vi "Octal Channel Engine.vi"(0 "Notifier Name":string) -> ()   [LabVIEW 2016]
uses:
  AOTF Controls/AOTF Actions.ctl
  AOTF Controls/AOTF Notifier Element.ctl
  Octal Channel Type Defs/Octal Channel AOTF Config.ctl
panel:
  in  "Wavelength (nm)":u16(ring)
  in  "Line On/Off":bool
  out "Controller Response":string
  in  "Blank All":bool
  in  "Quit":bool
  in  "Power (%)":dbl
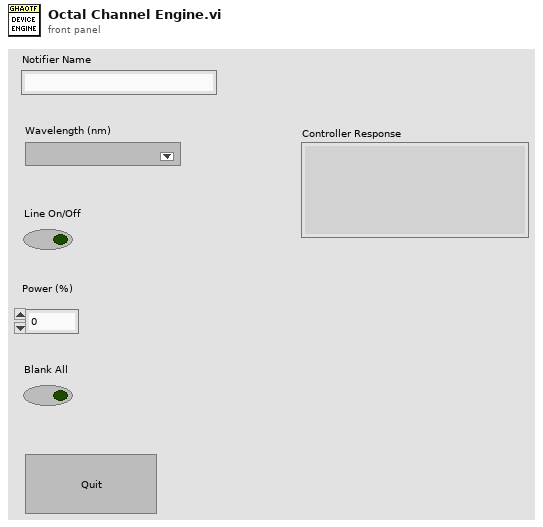
[diagram p1: front panel]
types:
  T1 = typedef "AOTF Notifier Element.ctl" = cluster{"AOTF Action":T2, "Laser Line":string, "Power (%)":dbl, "Beam Blank On/Off":bool, "Line On/Off":bool, "Error":errorcluster, "Wavelengths (nm)":string[]}
  T2 = typedef "AOTF Actions.ctl" = enum16{"Error Check", "Blank", "Line On/Off", "Set Power", "Status", "Quit"}
  T3 = typedef "Octal Channel AOTF Config.ctl" = cluster{"Wavelength (nm)":u16[], "Channel Number":u8[], "Frequency (MHz)":dbl[], "Max Power":u16[]}
  T4 = enum32{"Invalid", "Standard", "Closed", "Hidden", "Minimized", "Maximized"}
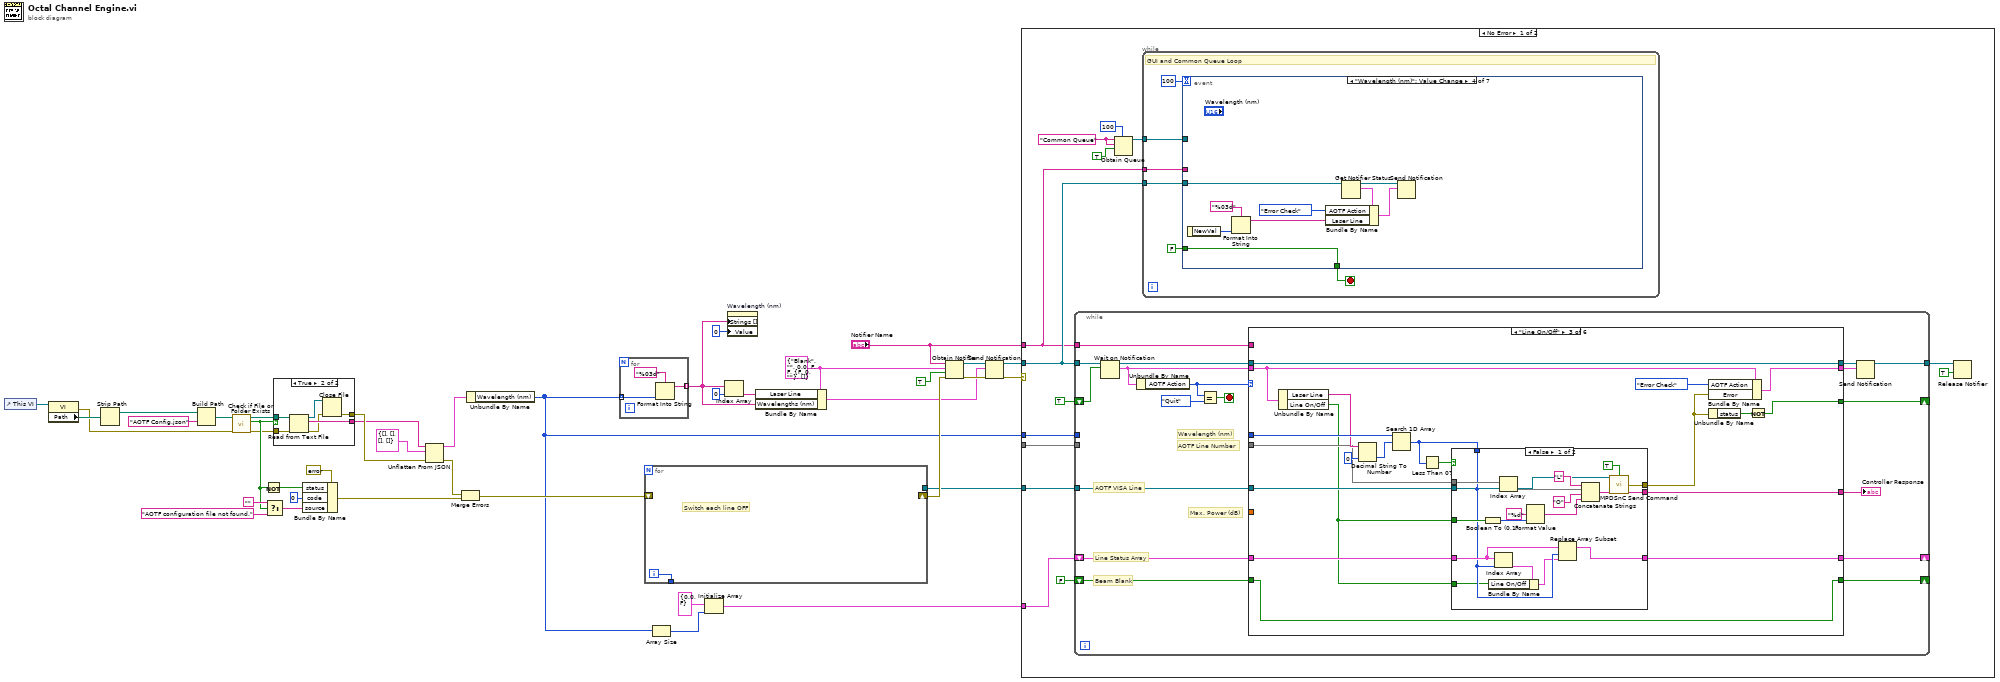
[diagram p0: block diagram]
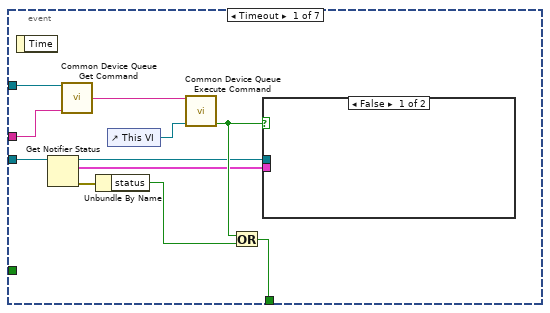
[diagram p2: hidden frame]
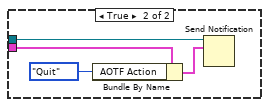
[diagram p3: hidden frame]
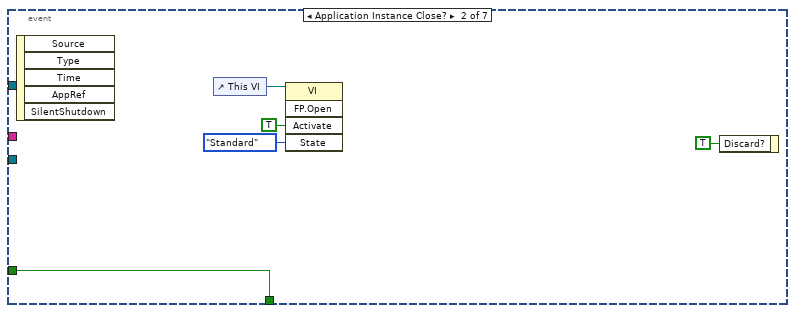
[diagram p4: hidden frame]
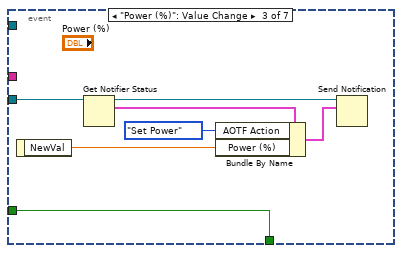
[diagram p5: hidden frame]
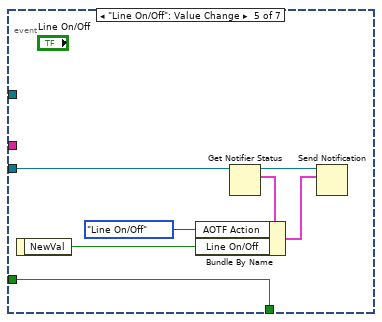
[diagram p6: hidden frame]
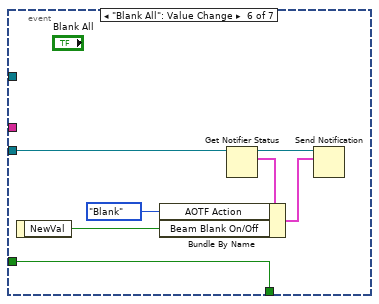
[diagram p7: hidden frame]
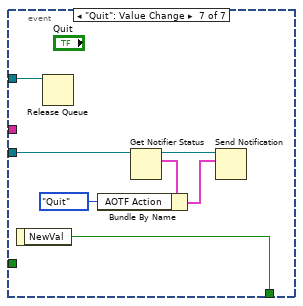
[diagram p8: hidden frame]
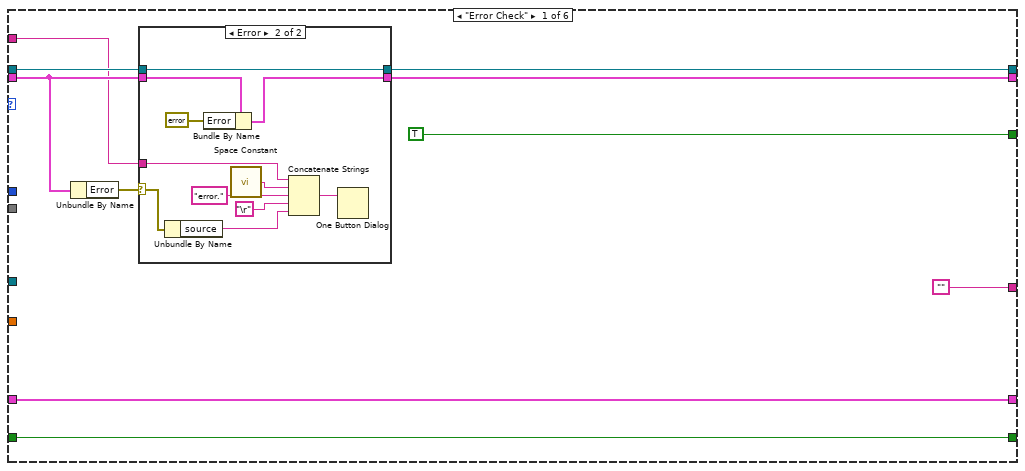
[diagram p9: hidden frame]
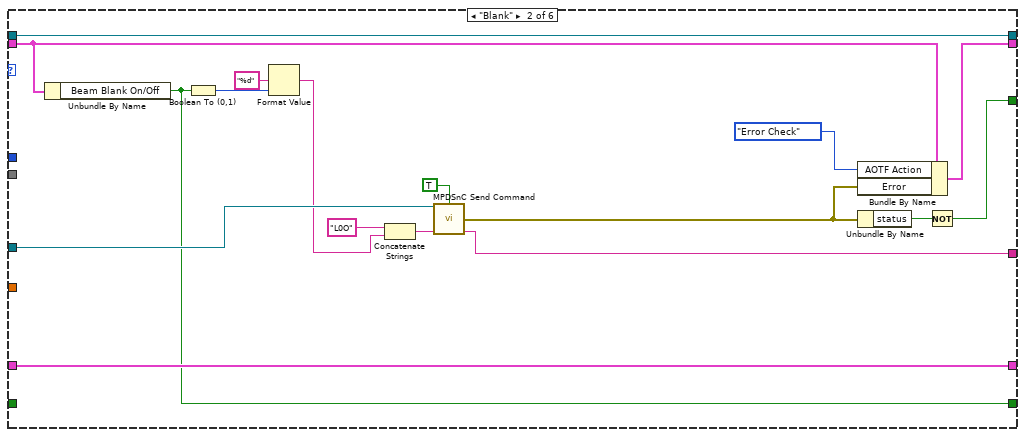
[diagram p11: hidden frame]
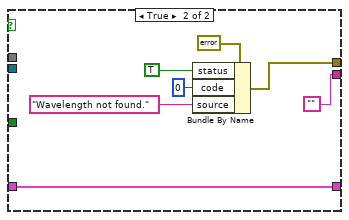
[diagram p12: hidden frame]
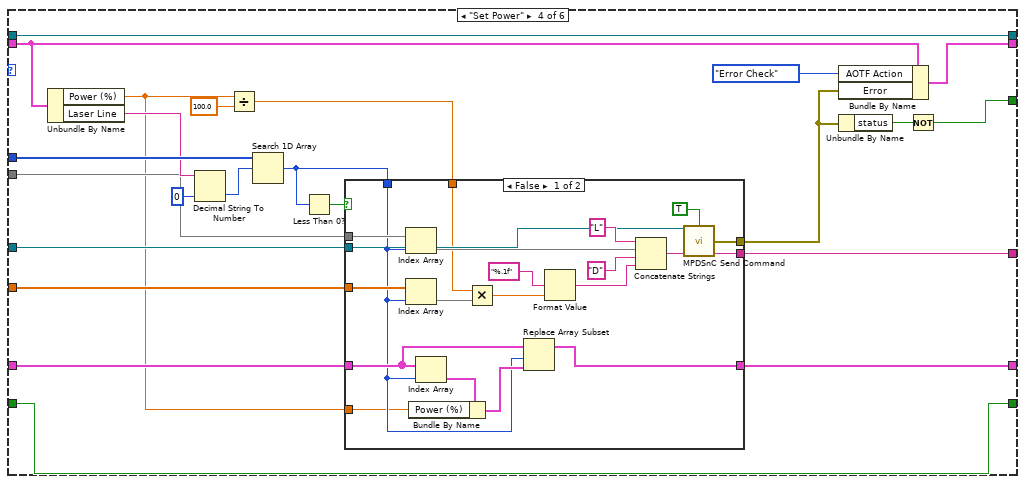
[diagram p13: hidden frame]
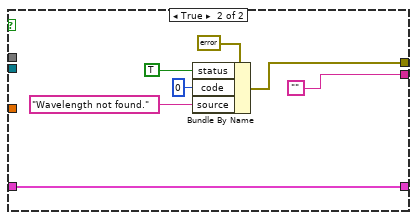
[diagram p14: hidden frame]
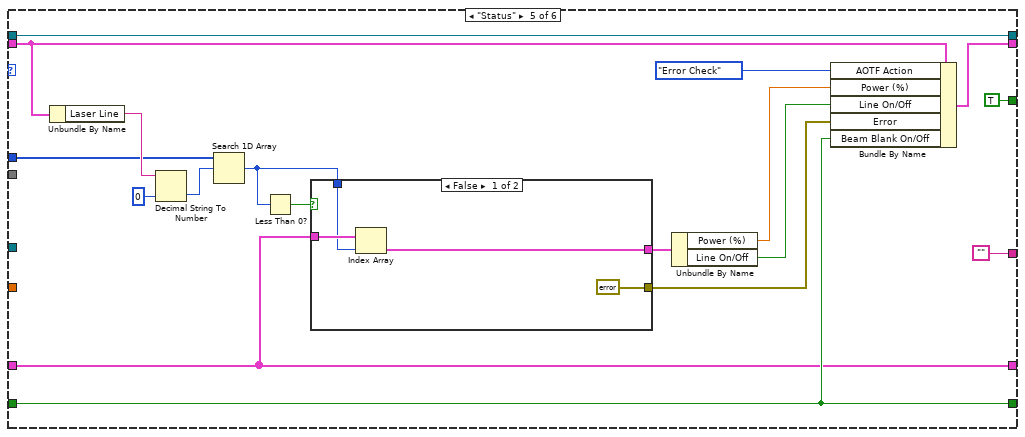
[diagram p15: hidden frame]
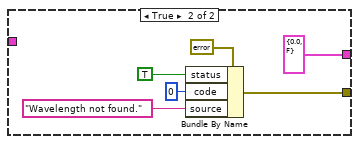
[diagram p16: hidden frame]
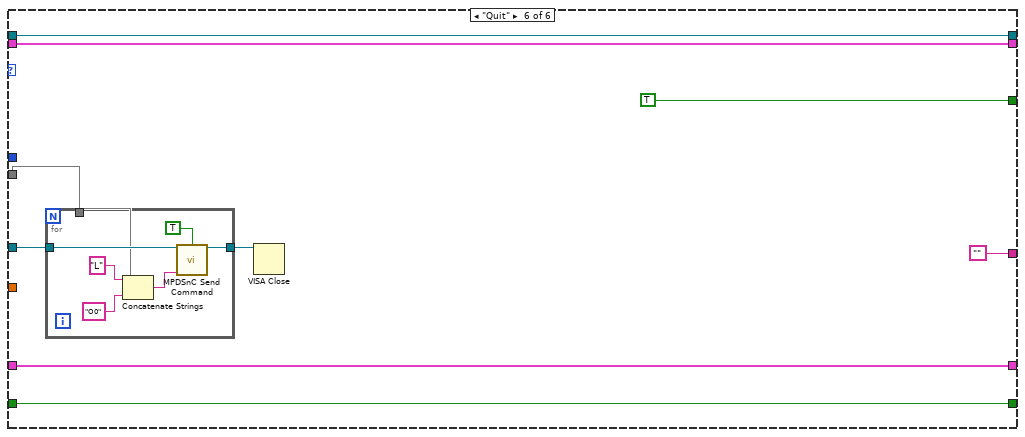
[diagram p17: hidden frame]
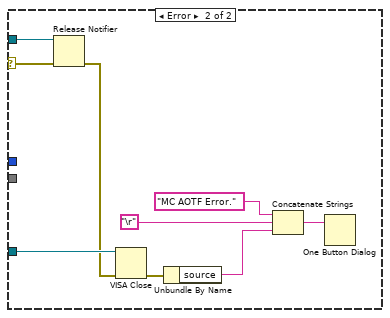
[diagram p18: hidden frame]
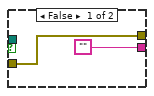
[diagram p19: hidden frame]
diagram:
  w10 = T1 {"AOTF Action"=enum."Blank", "Laser Line"="", "Power (%)"=0.0, "Beam Blank On/Off"=FALSE, "Line On/Off"=FALSE, "Error"={"status"=FALSE, "code"=0, "source"=""}, "Wavelengths (nm)"=[]} ("AOTFQueueCtrl")
  n1 = control-ref of="This VI"() -> (w40:refnum<vi>)
  n2 = property class="VI"(reference=w40) -> (error out=w27:errorcluster, "Path"=w39:path)  [unwired: 1 in, 1 out]
  n3 = Strip Path(path=w39) -> (stripped path=w38:path)  [unwired: 1 out]
  n4 = Build Path(base path=w38, name or relative path="AOTF Config.json") -> (appended path=w36:path)
  n5 = call <vilib>:"Check if File or Folder Exists.vi"("error in (no error)"=w27, "path"=w36) -> ("error out"=w26:errorcluster, "file or folder exists?"=w29:bool, "dup path"=w28:path)  [unwired: 7 in]
  n6 = Not(x=w29) -> (.not. x?=w34:bool)
  n7 = Select(t="", s=w29, f="AOTF configuration file not found." ("source")) -> (s? t:f=w30:string)
  n8 = case shown="True" w29 {
    tunnel: w28 -> [_ w48]
    tunnel: ["" w47] -> w22
    tunnel: w26 -> [w41 w45]
    tunnel: [w41 w43] -> w25
    frame False {
    }
    frame True {
      n9 = Read from Text File(file (use dialog)=w48, error in=w45) -> (refnum out=w46:refnum<file>, text=w47:string, error out=w44:errorcluster)  [unwired: 2 in, 1 out]
      n10 = Close File(refnum=w46, error in=w44) -> (error out=w43:errorcluster)  [unwired: 1 out]
    }
  }
  n11 = Bundle By Name(cluster=errorcluster {"status"=FALSE, "code"=0, "source"=""} ("Error"), "status"=w34, "code"=0, "source"=w30) -> (w23:errorcluster)
  n12 = Unflatten From JSON(JSON string=w22, type and defaults=T3 {"Wavelength (nm)"=[], "Channel Number"=[], "Frequency (MHz)"=[], "Max Power"=[]} ("AOTF Config"), error in (no error)=w25) -> (value=w7:T3, error out=w24:errorcluster)  [unwired: 4 in]
  n13 = Merge Errors(w24, w23) -> (w8:errorcluster)
  n14 = Unbundle By Name(w7) -> ("Wavelength (nm)"=w6:u16[])
  n15 = for {
    tunnel: w6 -> [w51] mode=indexing
    tunnel: [w50] -> w4 mode=indexing
    n16 = Format Into String(format string="%03d", w51) -> (resulting string=w50:string)  [unwired: 2 in, 1 out]
  }
  n17 = for {
    tunnel: [_] -> w17
    shift-right: [_] -> w20
    shift-left: w8 -> [_]
    tunnel: [w52] -> _
    i -> [w52]
    # "Switch each line OFF"
  }
  n18 = Array Size(array=w6) -> (size(s)=w5:i32)
  n19 = Initialize Array(cluster{"Power (%)":dbl, "Line On/Off":bool} {"Power (%)"=0.0, "Line On/Off"=FALSE} ("Line Staus Cluster"), w5) -> (w15:cluster{"Power (%)":dbl, "Line On/Off":bool}[])
  n20 = Index Array(array=w4, index=0) -> (element=w2:string)
  n21 = property on="Wavelength (nm)" class="Ring (strict)"("Strings []"=w4, "Value"=u16 0 ("index")) -> ()  [unwired: 2 in, 2 out]
  n22 = Bundle By Name(cluster=w10, "Laser Line"=w2, "Wavelengths (nm)"=w4) -> (w9:T1)
  n23 = Obtain Notifier(name (unnamed)="Notifier Name", notification data type=w10, create if not found? (T)=TRUE, error in (no error)=w20) -> (notifier out=w14:refnum<notifier>, error out=w13:errorcluster)  [unwired: 1 out]
  n24 = Send Notification(notification=w9, notifier=w14, error in (no error)=w13) -> (notifier out=w12:refnum<notifier>, error out=w11:errorcluster)
  n25 = case shown="No Error" w11 {
    selector: w11 -> [_ w336]
    tunnel: w12 -> [w62 w337]
    tunnel: "Notifier Name" -> [w58 _]
    tunnel: w6 -> [w57 _]
    tunnel: _ -> [w56 _]
    tunnel: w17 -> [w55 w331]
    tunnel: w15 -> [w54 _]
    frame No Error {
      w66 = "Common Queue" ("Unique Notifier Name")
      n26 = while {
        tunnel: w62 -> [w147]
        shift-right: [w138] -> _
        shift-left: TRUE ("ignore previous (F)") -> [w146]
        tunnel: [w137] -> w60
        tunnel: w58 -> [w136]
        tunnel: w57 -> [_]
        tunnel: w56 -> [_]
        tunnel: w55 -> [w135]
        shift-right: [w130] -> _
        shift-left: w54 -> [w133]
        shift-right: [w131] -> _
        shift-left: FALSE -> [w132]
        stop <- w141 stop-if-true
        # "Wavelength (nm)"
        # "AOTF Line Number"
        # "Line Status Array"
        # "Beam Blank"
        # "AOTF VISA Line"
        # "Max. Power (dB)"
        n27 = Wait on Notification(notifier=w147, ignore previous (F)=w146) -> (notifier out=w145:refnum<notifier>, notification=w144:T1)  [unwired: 2 in, 2 out]
        n28 = Unbundle By Name(w144) -> ("AOTF Action"=w143:T2)
        n29 = Equal?(x=w143, y=AOTF_Actions."Quit") -> (x = y?=w141:bool)
        n30 = case shown="\"Line On/Off\"" w143 {
          tunnel: w145 -> [w157 w187 w203 w256 w301 w321]
          tunnel: w144 -> [w155 w186 w205 w252 w296 w320]
          tunnel: [w153 w187 w203 w256 w301 w321] -> w140
          tunnel: [w152 w185 w204 w251 w292 w320] -> w139
          tunnel: [TRUE w182 w192 w250 TRUE TRUE] -> w138
          tunnel: w136 -> [w154 _ _ _ _ _]
          tunnel: _ -> [_ _ w200 w247 w297 _]
          tunnel: _ -> [_ _ w197 w243 _ w315]
          tunnel: _ -> [_ _ _ w240 _ _]
          tunnel: w135 -> [_ w180 w196 w239 _ w314]
          tunnel: ["" w173 w194 w238 "" ""] -> w134
          tunnel: w133 -> [w149 w172 w191 w237 w285 w317]
          tunnel: w132 -> [w148 _ w189 w234 w286 w316]
          tunnel: [w148 w171 w189 w234 w286 w316] -> w131
          tunnel: [w149 w172 w190 w235 w285 w317] -> w130
          frame "Error Check" {
            n31 = Unbundle By Name(w155) -> ("Error"=w156:errorcluster)
            n32 = case shown="Error" w156 {
              selector: w156 -> [_ w163]
              tunnel: w155 -> [w158 w167]
              tunnel: [w159 w165] -> w153
              tunnel: w157 -> [w159 w165]
              tunnel: w154 -> [_ w162]
              tunnel: [w158 w164] -> w152
              frame No Error {
              }
              frame Error {
                n33 = Unbundle By Name(w163) -> ("source"=w161:string)
                n34 = Bundle By Name(cluster=w167, "Error"=errorcluster {"status"=FALSE, "code"=0, "source"=""}) -> (w164:T1)
                n35 = call <vilib>:"Space Constant.vi"() -> ("String"=w170:string)
                n36 = Concatenate Strings(w162, w170, "error." ("string"), "\r", w161) -> (w168:string)
                n37 = One Button Dialog(message=w168) -> ()  [unwired: 1 in, 1 out]
              }
            }
          }
          frame "Blank" {
            n38 = Unbundle By Name(w186) -> ("Beam Blank On/Off"=w171:bool)
            n39 = Boolean To (0,1)(Boolean=w171) -> (0, 1=w176:i16)
            n40 = Format Value(format string="%d", value (0)=w176) -> (output string=w174:string)  [unwired: 1 in]
            n41 = Concatenate Strings("L0O", w174) -> (w177:string)
            n42 = call "MPDSnC Send Command.vi"("VISA Ref"=w180, "Wait for Reply?"=TRUE, "Command"=w177) -> ("Error Out"=w181:errorcluster, "Response"=w173:string)  [unwired: 10 in, 1 out]
            n43 = Bundle By Name(cluster=w186, "AOTF Action"=AOTF_Actions."Error Check", "Error"=w181) -> (w185:T1)
            n44 = Unbundle By Name(w181) -> ("status"=w183:bool)
            n45 = Not(x=w183) -> (.not. x?=w182:bool)
          }
          frame "Line On/Off" {
            n46 = Unbundle By Name(w205) -> ("Laser Line"=w199:string, "Line On/Off"=w188:bool)
            n47 = Decimal String To Number(string=w199, default (0L)=u16 0 ("default (0 I32)")) -> (number=w202:u16)  [unwired: 1 in, 1 out]
            n48 = Search 1D Array(1D array=w200, element=w202) -> (index of element=w195:i32)  [unwired: 1 in]
            n49 = Less Than 0?(x=w195) -> (x < 0?=w198:bool)
            n50 = case shown="False" w198 {
              tunnel: w197 -> [w226 _]
              tunnel: [w221 w229] -> w193
              tunnel: w195 -> [w211 _]
              tunnel: w196 -> [w219 _]
              tunnel: [w218 ""] -> w194
              tunnel: w188 -> [w215 _]
              tunnel: w191 -> [w213 w227]
              tunnel: [w212 w227] -> w190
              tunnel: w188 -> [w208 _]
              frame False {
                n51 = Boolean To (0,1)(Boolean=w215) -> (0, 1=w217:i16)
                n52 = Index Array(array=w213, index=w211) -> (element=w210:cluster{"Power (%)":dbl, "Line On/Off":bool})
                n53 = Bundle By Name(cluster=w210, "Line On/Off"=w208) -> (w209:cluster{"Power (%)":dbl, "Line On/Off":bool})
                n54 = Index Array(array=w226, index=w211) -> (element=w225)
                n55 = Format Value(format string="%d", value (0)=w217) -> (output string=w214:string)  [unwired: 1 in]
                n56 = Replace Array Subset(array=w213, new element=w209, index=w211) -> (w212:cluster{"Power (%)":dbl, "Line On/Off":bool}[])
                n57 = Concatenate Strings("L", w225, "O", w214) -> (w222:string)
                n58 = call "MPDSnC Send Command.vi"("VISA Ref"=w219, "Wait for Reply?"=TRUE, "Command"=w222) -> ("Error Out"=w221:errorcluster, "Response"=w218:string)  [unwired: 10 in, 1 out]
              }
              frame True {
                n59 = Bundle By Name(cluster=errorcluster {"status"=FALSE, "code"=0, "source"=""} ("error out"), "status"=TRUE, "code"=0, "source"="Wavelength not found.") -> (w229:errorcluster)
              }
            }
            n60 = Bundle By Name(cluster=w205, "AOTF Action"=AOTF_Actions."Error Check", "Error"=w193) -> (w204:T1)
            n61 = Unbundle By Name(w193) -> ("status"=w206:bool)
            n62 = Not(x=w206) -> (.not. x?=w192:bool)
          }
          frame "Set Power" {
            n63 = Unbundle By Name(w252) -> ("Power (%)"=w236:dbl, "Laser Line"=w246:string)
            n64 = Decimal String To Number(string=w246, default (0L)=u16 0 ("default (0 I32)")) -> (number=w248:u16)  [unwired: 1 in, 1 out]
            n65 = Divide(x=w236, y=100.0) -> (x/y=w242:dbl)
            n66 = Search 1D Array(1D array=w247, element=w248) -> (index of element=w244:i32)  [unwired: 1 in]
            n67 = Less Than 0?(x=w244) -> (x < 0?=w245:bool)
            n68 = case shown="False" w245 {
              tunnel: w243 -> [w277 _]
              tunnel: [w270 w280] -> w241
              tunnel: w244 -> [w260 _]
              tunnel: w242 -> [w259 _]
              tunnel: w240 -> [w274 _]
              tunnel: w239 -> [w265 _]
              tunnel: [w264 ""] -> w238
              tunnel: w237 -> [w261 w278]
              tunnel: w236 -> [w258 _]
              tunnel: [w257 w278] -> w235
              frame False {
                n69 = Index Array(array=w277, index=w260) -> (element=w276)
                n70 = Index Array(array=w274, index=w260) -> (element=w272)
                n71 = Index Array(array=w261, index=w260) -> (element=w263:cluster{"Power (%)":dbl, "Line On/Off":bool})
                n72 = Bundle By Name(cluster=w263, "Power (%)"=w258) -> (w262:cluster{"Power (%)":dbl, "Line On/Off":bool})
                n73 = Multiply(x=w259, y=w272) -> (x*y=w267:dbl)
                n74 = Replace Array Subset(array=w261, new element=w262, index=w260) -> (w257:cluster{"Power (%)":dbl, "Line On/Off":bool}[])
                n75 = Format Value(format string="%.1f", value (0)=w267) -> (output string=w266:string)  [unwired: 1 in]
                n76 = Concatenate Strings("L", w276, "D", w266) -> (w271:string)
                n77 = call "MPDSnC Send Command.vi"("VISA Ref"=w265, "Wait for Reply?"=TRUE, "Command"=w271) -> ("Error Out"=w270:errorcluster, "Response"=w264:string)  [unwired: 10 in, 1 out]
              }
              frame True {
                n78 = Bundle By Name(cluster=errorcluster {"status"=FALSE, "code"=0, "source"=""} ("error out"), "status"=TRUE, "code"=0, "source"="Wavelength not found.") -> (w280:errorcluster)
              }
            }
            n79 = Bundle By Name(cluster=w252, "AOTF Action"=AOTF_Actions."Error Check", "Error"=w241) -> (w251:T1)
            n80 = Unbundle By Name(w241) -> ("status"=w253:bool)
            n81 = Not(x=w253) -> (.not. x?=w250:bool)
          }
          frame "Status" {
            n82 = Unbundle By Name(w296) -> ("Laser Line"=w298:string)
            n83 = Decimal String To Number(string=w298, default (0L)=u16 0 ("default (0 I32)")) -> (number=w299:u16)  [unwired: 1 in, 1 out]
            n84 = Search 1D Array(1D array=w297, element=w299) -> (index of element=w294:i32)  [unwired: 1 in]
            n85 = Less Than 0?(x=w294) -> (x < 0?=w295:bool)
            n86 = case shown="False" w295 {
              tunnel: w285 -> [w306 _]
              tunnel: [errorcluster {"status"=FALSE, "code"=0, "source"=""} ("error out") w308] -> w290
              tunnel: w294 -> [w305 _]
              tunnel: [w304 cluster{"Power (%)":dbl, "Line On/Off":bool} {"Power (%)"=0.0, "Line On/Off"=FALSE} ("Line Staus Cluster")] -> w289
              frame False {
                n87 = Index Array(array=w306, index=w305) -> (element=w304:cluster{"Power (%)":dbl, "Line On/Off":bool})
              }
              frame True {
                n88 = Bundle By Name(cluster=errorcluster {"status"=FALSE, "code"=0, "source"=""} ("error out"), "status"=TRUE, "code"=0, "source"="Wavelength not found.") -> (w308:errorcluster)
              }
            }
            n89 = Unbundle By Name(w289) -> ("Power (%)"=w288:dbl, "Line On/Off"=w287:bool)
            n90 = Bundle By Name(cluster=w296, "AOTF Action"=AOTF_Actions."Error Check", "Power (%)"=w288, "Line On/Off"=w287, "Error"=w290, "Beam Blank On/Off"=w286) -> (w292:T1)
          }
          frame "Quit" {
            n91 = for {
              tunnel: w314 -> [w327]
              tunnel: w315 -> [w325]
              tunnel: [w322] -> w313
              n92 = Concatenate Strings("L", w325, "O0" ("string")) -> (w324:string)
              n93 = call "MPDSnC Send Command.vi"("VISA Ref"=w327, "Wait for Reply?"=TRUE, "Command"=w324) -> ("VISA Ref Out"=w322:refnum<visa-resource-name>)  [unwired: 10 in, 2 out]
            }
            n94 = VISA Close(VISA resource name=w313) -> ()  [unwired: 1 in, 1 out]
          }
        }
        "Controller Response" <- w134
        n95 = Send Notification(notification=w139, notifier=w140) -> (notifier out=w137:refnum<notifier>)  [unwired: 1 in, 1 out]
      }
      n96 = Obtain Queue(max queue size (-1, unlimited)=100, name (unnamed)=w66, element data type=w66, create if not found? (T)=TRUE) -> (queue out=w63:refnum<queue>)  [unwired: 1 in, 2 out]
      n97 = while {
        tunnel: w63 -> [w71]
        tunnel: w58 -> [w69]
        tunnel: w62 -> [w70]
        stop <- w68 stop-if-true
        # "GUI and Common Queue Loop"
        n98 = event shown="[3] \"Wavelength (nm)\": Value Change" {
          selector: _ -> [_ _ _ _ _ _ _]
          dyn-events: _ -> [_ _ _ _ _ _ _]
          timeout: 100 -> [_ _ _ _ _ _ _]
          tunnel: w71 -> [w78 _ _ _ _ _ w129]
          tunnel: w70 -> [w74 _ w95 w105 w111 w121 w128]
          tunnel: w69 -> [w77 _ _ _ _ _ _]
          tunnel: [w76 w92 w99 w108 w115 w122 w126] -> w68
          tunnel: FALSE -> [_ w92 w99 w108 w115 w122 _]
          event Timeout {
            n99 = event-data() -> ()  [unwired: 1 in, 1 out]
            n100 = Get Notifier Status(notifier=w74) -> (notifier out=w73:refnum<notifier>, current notification=w75:T1, error out=w83:errorcluster)  [unwired: 1 in, 2 out]
            n101 = call "Common Device Queue Get Command.vi"("Common Queue"=w78, "Notifier Name"=w77) -> ("Command"=w82:string)  [unwired: 12 in, 1 out]
            n102 = Unbundle By Name(w83) -> ("status"=w80:bool)
            n103 = control-ref of="This VI"() -> (w81:refnum<vi>)
            n104 = call "Common Device Queue Execute Command.vi"("Common Command"=w82, "VI Refnum"=w81) -> ("Quit?"=w79:bool)  [unwired: 12 in, 1 out]
            n105 = Or(x=w79, y=w80) -> (x .or. y?=w76:bool)
            n106 = case shown="False" w79 {
              tunnel: w73 -> [_ w87]
              tunnel: w75 -> [_ w86]
              frame False {
              }
              frame True {
                n107 = Bundle By Name(cluster=w86, "AOTF Action"=AOTF_Actions."Quit") -> (w85:T1)
                n108 = Send Notification(notification=w85, notifier=w87) -> ()  [unwired: 1 in, 2 out]
              }
            }
          }
          event Application Instance Close? {
            n109 = event-data() -> ()  [unwired: 1 in, 5 out]
            n110 = control-ref of="This VI"() -> (w89:refnum<vi>)
            n111 = invoke class="VI" method="FP.Open"(reference=w89, "Activate"=TRUE ("Activate?"), "State"=T4."Standard") -> ()  [unwired: 2 in, 5 out]
            n112 = event-data("Discard?"=TRUE) -> ()  [unwired: 1 in, 1 out]
          }
          event "Power (%)": Value Change {
            n113 = event-data() -> ("NewVal"=w97:dbl)  [unwired: 1 in]
            n114 = Get Notifier Status(notifier=w95) -> (notifier out=w93:refnum<notifier>, current notification=w94:T1)  [unwired: 1 in, 3 out]
            n115 = Bundle By Name(cluster=w94, "AOTF Action"=AOTF_Actions."Set Power", "Power (%)"=w97) -> (w96:T1)
            n116 = Send Notification(notification=w96, notifier=w93) -> ()  [unwired: 1 in, 2 out]
          }
          event "Wavelength (nm)": Value Change {
            n117 = event-data() -> ("NewVal"=w101:u16)  [unwired: 1 in]
            n118 = Format Into String(format string="%03d", w101) -> (resulting string=w100:string)  [unwired: 2 in, 1 out]
            n119 = Get Notifier Status(notifier=w105) -> (notifier out=w103:refnum<notifier>, current notification=w104:T1)  [unwired: 1 in, 3 out]
            n120 = Bundle By Name(cluster=w104, "AOTF Action"=AOTF_Actions."Error Check", "Laser Line"=w100) -> (w106:T1)
            n121 = Send Notification(notification=w106, notifier=w103) -> ()  [unwired: 1 in, 2 out]
          }
          event "Line On/Off": Value Change {
            n122 = event-data() -> ("NewVal"=w110:bool)  [unwired: 1 in]
            n123 = Get Notifier Status(notifier=w111) -> (notifier out=w114:refnum<notifier>, current notification=w113:T1)  [unwired: 1 in, 3 out]
            n124 = Bundle By Name(cluster=w113, "AOTF Action"=AOTF_Actions."Line On/Off", "Line On/Off"=w110) -> (w109:T1)
            n125 = Send Notification(notification=w109, notifier=w114) -> ()  [unwired: 1 in, 2 out]
          }
          event "Blank All": Value Change {
            n126 = event-data() -> ("NewVal"=w117:bool)  [unwired: 1 in]
            n127 = Get Notifier Status(notifier=w121) -> (notifier out=w120:refnum<notifier>, current notification=w119:T1)  [unwired: 1 in, 3 out]
            n128 = Bundle By Name(cluster=w119, "AOTF Action"=AOTF_Actions."Blank", "Beam Blank On/Off"=w117) -> (w116:T1)
            n129 = Send Notification(notification=w116, notifier=w120) -> ()  [unwired: 1 in, 2 out]
          }
          event "Quit": Value Change {
            n130 = event-data() -> ("NewVal"=w126:bool)  [unwired: 1 in]
            n131 = Release Queue(queue=w129) -> ()  [unwired: 2 in, 3 out]
            n132 = Get Notifier Status(notifier=w128) -> (notifier out=w127:refnum<notifier>, current notification=w125:T1)  [unwired: 1 in, 3 out]
            n133 = Bundle By Name(cluster=w125, "AOTF Action"=AOTF_Actions."Quit") -> (w123:T1)
            n134 = Send Notification(notification=w123, notifier=w127) -> ()  [unwired: 1 in, 2 out]
          }
        }
      }
      n135 = Release Notifier(notifier=w60, force destroy? (F)=TRUE) -> ()  [unwired: 1 in, 3 out]
    }
    frame Error {
      n136 = Release Notifier(notifier=w337, error in (no error)=w336) -> (error out=w330:errorcluster)  [unwired: 1 in, 2 out]
      n137 = VISA Close(VISA resource name=w331, error in (no error)=w330) -> (error out=w329:errorcluster)
      n138 = Unbundle By Name(w329) -> ("source"=w333:string)
      n139 = Concatenate Strings("MC AOTF Error.", "\r", w333) -> (w332:string)
      n140 = One Button Dialog(message=w332) -> ()  [unwired: 1 in, 1 out]
    }
  }
